vi "Network Read.vi"(8 "error in (no error)":errorcluster, 9 "Status_Cluster_in":T1={"simTime"=0.0, "simFrame"=0.0, "Connection Status"=enum."Disconnected", "Connection Command"=enum."Disconnect", "Last Error"=0, "Case selection"=enum."Connecting"}, 10 "RDB References in":T7 {"RDB Send Reference"."RDB Data"."payload" format="%x"; "RDB Send Reference"."RDB Data"."timestamp" format="%<%.7X\n%x>T"; "RDB Send Reference"."RDB Data"."type" items=["FlexRay Data"=32, "FlexRay Null"=33, "FlexRay Symbol"=34, "Log Trigger"=225, "Start Trigger"=226]; "RDB Send Reference"."RDB Data"."cycle count" max=63 step=1; "RDB Receive Reference"."RDB Data"."payload" format="%x"; "RDB Receive Reference"."RDB Data"."timestamp" format="%<%.7X\n%x>T"; "RDB Receive Reference"."RDB Data"."type" items=["FlexRay Data"=32, "FlexRay Null"=33, "FlexRay Symbol"=34, "Log Trigger"=225, "Start Trigger"=226]; "RDB Receive Reference"."RDB Data"."cycle count" max=63 step=1}, 11 "Settings":T4={"UDP Receiver"=refnum, "UDP Sender"=refnum, "Valid Packet"=FALSE, "TCP"=refnum, "Network Settings"={"IP adress"="127.0.0.1", "RDB"={"Protocol"=enum."UDP", "Tx Port"=48270, "Rx Port"=10, "Buffer Size"=204800, "Timeout"=10}, "SCP"={"Protocol"=enum."TCP", "Tx Port"=48191, "Rx Port"=48191, "Buffer Size"=204800, "Timeout"=10}}, "vclient"=path ""}) -> (0 "error out":errorcluster, 1 "Status_Cluster_out":T1={"simTime"=0.0, "simFrame"=0.0, "Connection Status"=enum."Disconnected", "Connection Command"=enum."Disconnect", "Last Error"=0, "Case selection"=enum."Connecting"}, 2 "RDB References out":T7 {"RDB Send Reference"."RDB Data"."payload" format="%x"; "RDB Send Reference"."RDB Data"."timestamp" format="%<%.7X\n%x>T"; "RDB Send Reference"."RDB Data"."type" items=["FlexRay Data"=32, "FlexRay Null"=33, "FlexRay Symbol"=34, "Log Trigger"=225, "Start Trigger"=226]; "RDB Send Reference"."RDB Data"."cycle count" max=63 step=1; "RDB Receive Reference"."RDB Data"."payload" format="%x"; "RDB Receive Reference"."RDB Data"."timestamp" format="%<%.7X\n%x>T"; "RDB Receive Reference"."RDB Data"."type" items=["FlexRay Data"=32, "FlexRay Null"=33, "FlexRay Symbol"=34, "Log Trigger"=225, "Start Trigger"=226]; "RDB Receive Reference"."RDB Data"."cycle count" max=63 step=1}, 3 "Settings":T4={"UDP Receiver"=refnum, "UDP Sender"=refnum, "Valid Packet"=FALSE, "TCP"=refnum, "Network Settings"={"IP adress"="127.0.0.1", "RDB"={"Protocol"=enum."UDP", "Tx Port"=48270, "Rx Port"=10, "Buffer Size"=204800, "Timeout"=10}, "SCP"={"Protocol"=enum."TCP", "Tx Port"=48191, "Rx Port"=48191, "Buffer Size"=204800, "Timeout"=10}}, "vclient"=path ""}, 4 "Packet Size":i32, 5 "RDB Receive Reference.RDB Signals":dbl[](array[numeric]))   [LabVIEW 2020, in "Vires VTD Engine.lvlib"]
uses:
  Vires VTD Engine.lvlib
  RDB/RDB References.ctl
  RDB/RDB Reference.ctl
  <vilib>/xnet/xnet.llb/XNET Frame FlexRay.ctl
  <vilib>/xnet/xnet.llb/XNET Frame Type FlexRay.ctl
  Type/Settings.ctl
  Shared/Network Settings.ctl
  Shared/Protocol.ctl
  Type/Status_Cluster.ctl
  Type/ConnectionStatus.ctl
  Type/CaseSelection.ctl
  RDB/RDB.lvlib
  Shared/Vires VTD Shared.lvlib
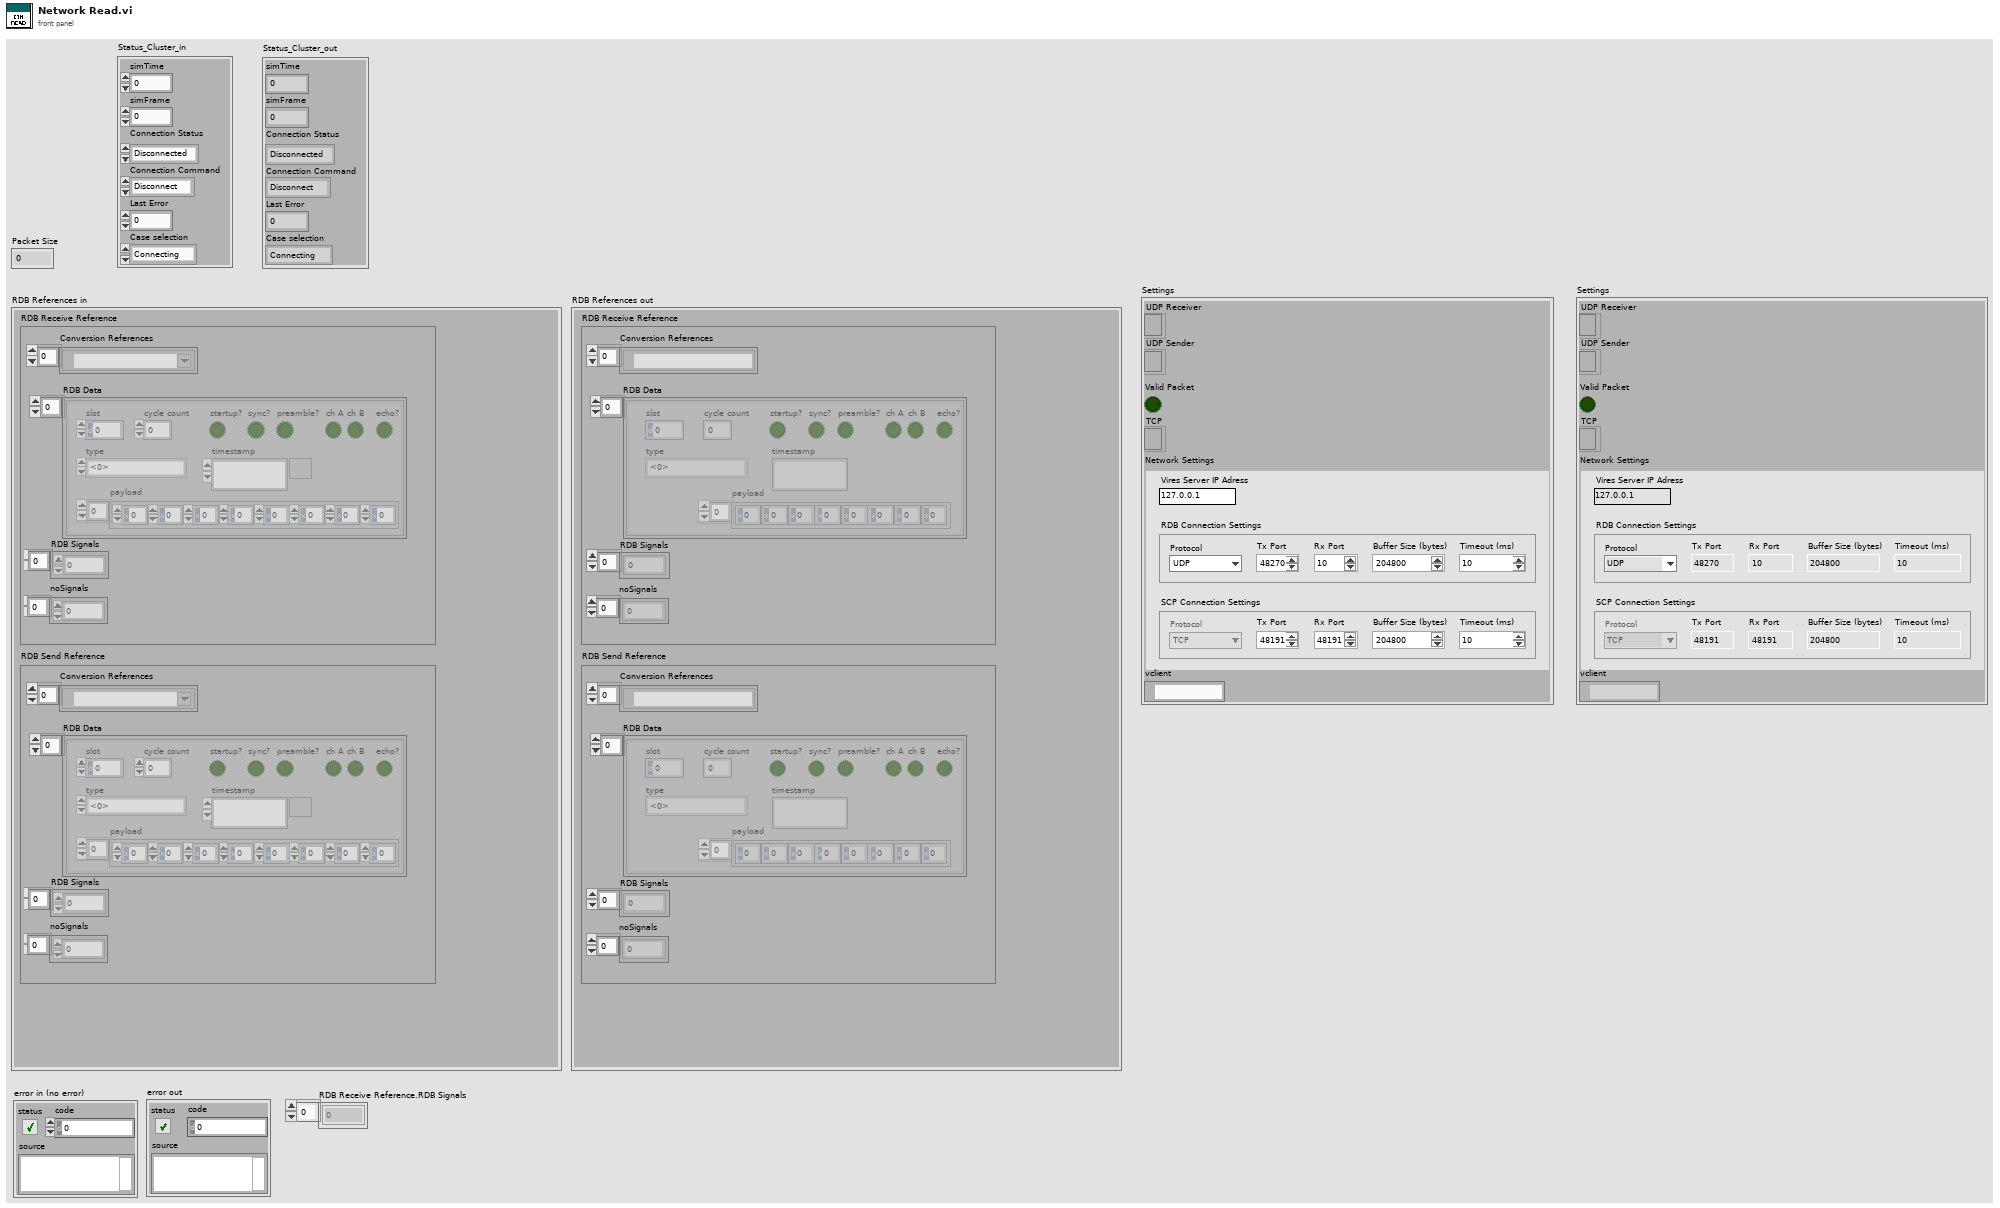
[diagram p1: front panel]
types:
  T1 = typedef "Vires VTD Engine.lvlib/Status_Cluster.ctl" = cluster{"simTime":dbl, "simFrame":dbl, "Connection Status":T2, "Connection Command":enum16{"Disconnect", "Connect"}, "Last Error":i32, "Case selection":T3}
  T2 = typedef "Vires VTD Engine.lvlib/ConnectionStatus.ctl" = enum16{"Disconnected", "Connected"}
  T3 = typedef "Vires VTD Engine.lvlib/CaseSelection.ctl" = enum32{"Idle", "Connecting", "Disconnecting", "Read/Write"}
  T4 = typedef "Vires VTD Engine.lvlib/Settings.ctl" = cluster{"UDP Receiver":refnum<k16>, "UDP Sender":refnum<k16>, "Valid Packet":bool, "TCP":refnum<k5>, "Network Settings":T5, "vclient":path}
  T5 = typedef "Vires VTD Shared.lvlib/Network Settings.ctl" = cluster{"IP adress":string, "RDB":cluster{"Protocol":T6, "Tx Port":u16, "Rx Port":u16, "Buffer Size":i32, "Timeout":u16}, "SCP":cluster{"Protocol":T6, "Tx Port":u16, "Rx Port":u16, "Buffer Size":i32, "Timeout":u16}}
  T6 = typedef "Vires VTD Shared.lvlib/Protocol.ctl" = enum16{"UDP", "TCP"}
  T7 = typedef "RDB.lvlib/RDB References.ctl" = cluster{"RDB Receive Reference":T8, "RDB Send Reference":T8}
  T8 = typedef "RDB.lvlib/RDB Reference.ctl" = cluster{"Conversion References":refnum<k21>[], "RDB Data":T9[], "RDB Signals":dbl[], "noSignals":i32[]}
  T9 = typedef "XNET Frame FlexRay.ctl" = cluster{"timestamp":timestamp, "payload":u8[], "slot":u16, "type":T10, "cycle count":u8, "startup?":bool, "sync?":bool, "preamble?":bool, "ch A":bool, "ch B":bool, "echo?":bool}
  T10 = typedef "XNET Frame Type FlexRay.ctl" = u8
  T11 = enum16{"Standard", "Buffered", "CRLF", "Immediate"}
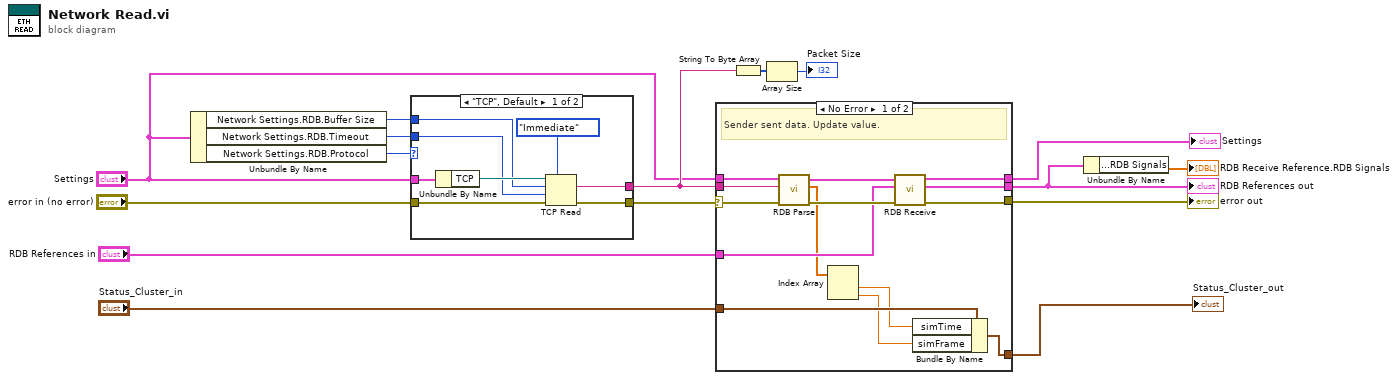
[diagram p0: block diagram]
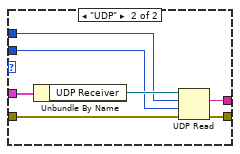
[diagram p2: hidden frame]
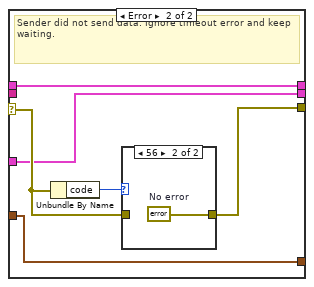
[diagram p3: hidden frame]
diagram:
  n1 = Unbundle By Name("Settings") -> ("Network Settings.RDB.Buffer Size"=w4:i32, "Network Settings.RDB.Timeout"=w5:u16, "Network Settings.RDB.Protocol"=w6:T6)
  n2 = case shown="\"TCP\", Default" w6 {
    tunnel: "error in (no error)" -> [w23 w31]
    tunnel: [w22 w30] -> w15
    tunnel: "Settings" -> [w24 w28]
    tunnel: [w21 w27] -> w10
    tunnel: w4 -> [w17 w26]
    tunnel: w5 -> [w18 w25]
    frame "TCP", Default {
      n3 = Unbundle By Name(w24) -> ("TCP"=w20:refnum<k5>)
      n4 = TCP Read(connection ID=w20, bytes to read=w17, error in (no error)=w23, 7:T11."Immediate" ("mode (standard)"), 9:w18) -> (data out=w21:string, error out=w22:errorcluster)  [unwired: 1 out]
    }
    frame "UDP" {
      n5 = Unbundle By Name(w28) -> ("UDP Receiver"=w29:refnum<k16>)
      n6 = UDP Read(connection ID=w29, max size (548)=w26, timeout ms (25000)=w25, 8:w31) -> (data out=w27:string, error out=w30:errorcluster)  [unwired: 3 out]
    }
  }
  n7 = case shown="No Error" w15 {
    selector: w15 -> [w45 w50]
    tunnel: [w42 w49] -> w13
    tunnel: "RDB References in" -> [w37 w48]
    tunnel: [w41 w48] -> w12
    tunnel: w10 -> [w43 _]
    tunnel: "Settings" -> [w40 w47]
    tunnel: [w38 w47] -> w7
    tunnel: "Status_Cluster_in" -> [w36 w46]
    tunnel: [w33 w46] -> w1
    frame No Error {
      # "Sender sent data. Update value."
      n8 = call "RDB Parse.vi"("error in (no error)"=w45, "RDB Message"=w43, "Settings"=w40) -> ("error out"=w44:errorcluster, "Status"=w34:dbl[], "Settings"=w39:T4)  [unwired: 6 in]
      n9 = Index Array(array=w34) -> (element #1=w35:dbl, element #2=w32:dbl)  [unwired: 2 in]
      n10 = call "RDB Receive.vi"("error in (no error)"=w44, "RDB Reference in"=w37, "Settings"=w39) -> ("error out"=w42:errorcluster, "RDB Reference out"=w41:T7, "Settings"=w38:T4)  [unwired: 6 in]
      n11 = Bundle By Name(cluster=w36, "simTime"=w35, "simFrame"=w32) -> (w33:T1)
    }
    frame Error {
      # "Sender did not send data. Ignore timeout error and keep waiting."
      n12 = Unbundle By Name(w50) -> ("code"=w51:i32)
      n13 = case shown="56" w51 {
        tunnel: w50 -> [w52 _]
        tunnel: [w52 w53] -> w49
        frame Default {
        }
        frame 56 {
          w53 = errorcluster {"status"=FALSE, "code"=0, "source"=""}  # No error
        }
      }
    }
  }
  "RDB References out" <- w12
  "error out" <- w13
  "Settings" <- w7
  "Status_Cluster_out" <- w1
  n14 = String To Byte Array(string=w10) -> (unsigned byte array=w9:u8[])
  n15 = Array Size(array=w9) -> (size(s)=→"Packet Size":i32)
  n16 = Unbundle By Name(w12) -> ("RDB Receive Reference.RDB Signals"=→"RDB Receive Reference.RDB Signals":dbl[])
